vi "Refresh Alarms.vi"(8 "error in":errorcluster, 9 "Source":string, 10 "Code":string, 11 "Fault Handler in":refnum<class "Fault Handler.lvclass">) -> (0 "error out":errorcluster, 3 "Fault Handler out":refnum<class "Fault Handler.lvclass">)   [LabVIEW 2019, in "Fault Handler.lvlib" / "Fault Handler.lvclass"]
doc: "Called when error data is provided. \nThis routine checks the active error data to confirm if the error is already active: \n\n<b>Error Already Active</b>\nThe routine skips all additional steps and calls <b>Refresh Display</b>\n\n<b>Error Not Active</b>\nThe Error is added to the active error list and constructs an error log record\nThe log record is written to the error log output file and appended to the Error history indicator\nThe routine calls <b>Refresh Display</b>\nThe routine calls <b>Terminate Automation</b>"
uses:
  Project/Fault Handler.lvclass
  Project/Fault Handler.lvclass/Fault Handler.ctl
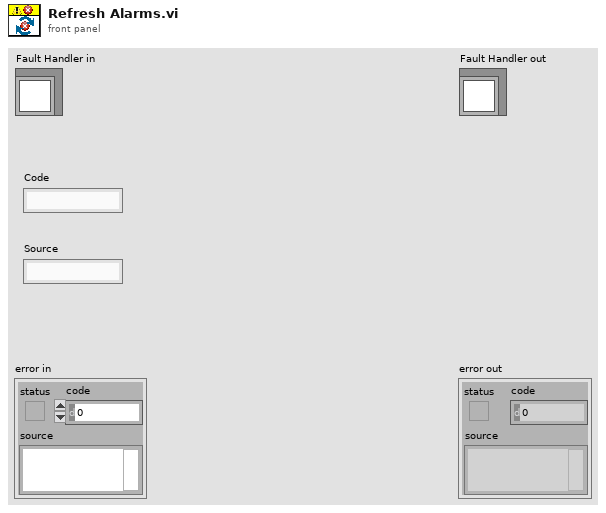
[diagram p1: front panel]
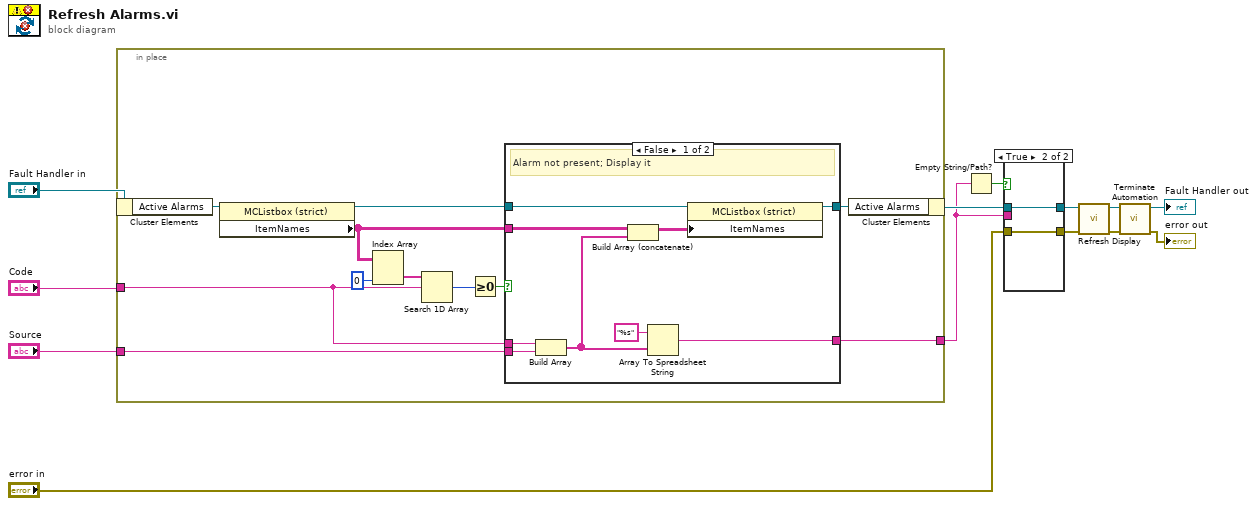
[diagram p0: block diagram]
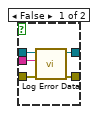
[diagram p2: hidden frame]
diagram:
  n1 = in-place {
    in-place-border: "Code" -> [w17]
    in-place-border: "Source" -> [w16]
    in-place-border: [w14] -> w6
    n2 = in-place-cluster #1("Fault Handler in") -> ("Active Alarms"=w24:refnum<vi>)
    n3 = property class="MCListbox (strict)"(reference=w24) -> (reference out=w19:refnum<vi>, "ItemNames"=w15:string[][])  [unwired: 1 in, 1 out]
    n4 = Index Array(array=w15, index (col)=0) -> (element=w22:string[])  [unwired: 1 in]
    n5 = Search 1D Array(1D array=w22, element=w17) -> (index of element=w21:i32)  [unwired: 1 in]
    n6 = Greater Or Equal To 0?(x=w21) -> (x >= 0?=w20:bool)
    n7 = case shown="False" w20 {
      tunnel: w19 -> [w33 w34]
      tunnel: [w32 w34] -> w18
      tunnel: w17 -> [w31 _]
      tunnel: w16 -> [w30 _]
      tunnel: w15 -> [w29 _]
      tunnel: [w25 _] -> w14
      frame False {
        # "Alarm not present; Display it"
        n8 = Build Array(w31, w30) -> (w27:string[])
        n9 = Build Array (concatenate)(w29, w27) -> (w28:string[][])
        n10 = Array To Spreadsheet String(array=w27, 3:"%s" ("format string")) -> (spreadsheet string=w25:string)  [unwired: 1 in]
        n11 = property class="MCListbox (strict)"(reference=w33, "ItemNames"=w28) -> (reference out=w32:refnum<vi>)  [unwired: 1 in, 1 out]
      }
      frame True {
        # "Alarm Already Present; do not duplicate"
      }
    }
    n12 = in-place-cluster #1("Active Alarms"=w18) -> (w7:refnum<class "Fault Handler.lvclass">)
  }
  n13 = Empty String/Path?(string/path=w6) -> (empty?=w5:bool)
  n14 = case shown="True" w5 {
    tunnel: w7 -> [w39 w41]
    tunnel: [w38 w41] -> w10
    tunnel: [w37 w40] -> w9
    tunnel: "error in" -> [w36 w40]
    tunnel: w6 -> [w35 _]
    frame False {
      n15 = call "Log Error Data.vi"("error in"=w36, "Error Data"=w35, "Fault Handler in"=w39) -> ("error out"=w37:errorcluster, "Fault Handler out"=w38:refnum<class "Fault Handler.lvclass">)  [unwired: 7 in]
    }
    frame True {
    }
  }
  n16 = call "Refresh Display.vi"("error in"=w9, "Fault Handler in"=w10) -> ("error out"=w4:errorcluster, "Fault Handler out"=w3:refnum<class "Fault Handler.lvclass">)  [unwired: 8 in]
  n17 = call "Terminate Automation.vi"("error in"=w4, "Fault Handler in"=w3) -> ("error out"=→"error out":errorcluster, "Fault Handler out"=→"Fault Handler out":refnum<class "Fault Handler.lvclass">)  [unwired: 8 in]
